vi "Init.vi"(0 "Data3D in":refnum<class "Data3D.lvclass">, 11 "error in (no error)":errorcluster) -> (4 "Data3D out":refnum<class "Data3D.lvclass">, 15 "error out":errorcluster)   [LabVIEW 2014, in "Data3D.lvclass"]
uses:
  Data3D.lvclass
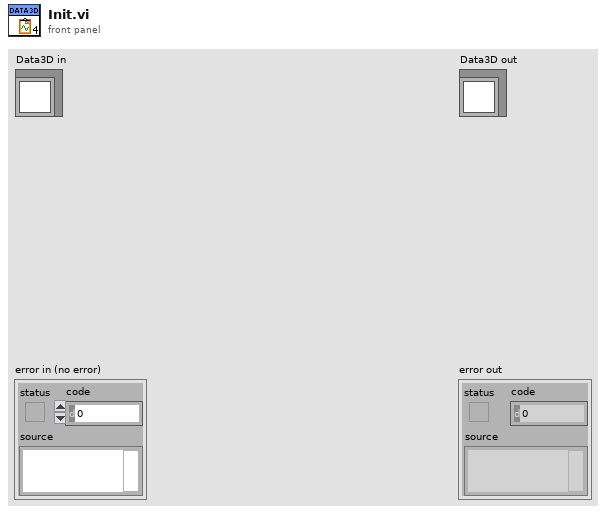
[diagram p1: front panel]
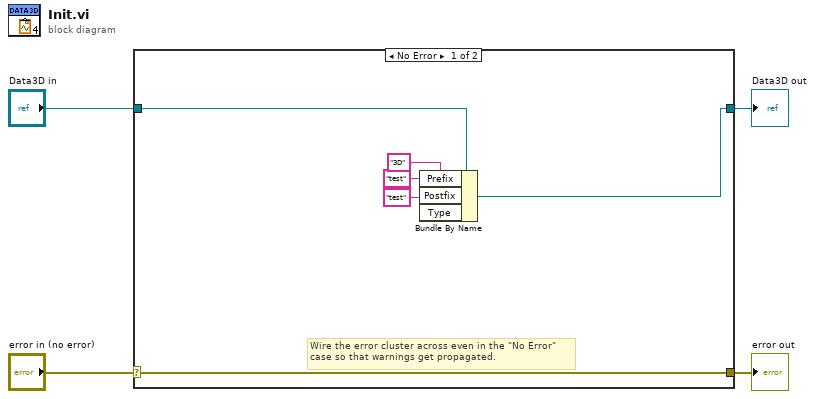
[diagram p0: block diagram]
diagram:
  n1 = case shown="No Error" "error in (no error)" {
    selector: "error in (no error)" -> [w10 w12]
    tunnel: [w10 w12] -> w3
    tunnel: [w8 w11] -> w1
    tunnel: "Data3D in" -> [w9 w11]
    frame No Error {
      # "Wire the error cluster across even in the \"No Error\"\ncase so that warnings get propagated."
      n2 = Bundle By Name(cluster=w9, "Prefix"="test", "Postfix"="test", "Type"="3D") -> (w8:refnum<class "Data3D.lvclass">)
    }
    frame Error {
    }
  }
  "error out" <- w3
  "Data3D out" <- w1
